vi "TCC_LIBRA.vi"() -> ()   [LabVIEW 2010]
doc: "Use this template to build a standard state machine design pattern. Each state executes code and determines which state to transition to. Contrast this design pattern with the User Interface Event Handler pattern, in which code executes in response to user actions. Contrast this design pattern also with the Queued Message Handler pattern, in which each message handling code can queue zero or more new messages."
uses:
  LV/TCC_03_02_2016/TCC_01_02_15.ctl
  <vilib>/Instr/_visa.llb/VISA Configure Serial Port (Instr).vi
  <vilib>/Utility/file.llb/Write To Spreadsheet File (DBL).vi
  <vilib>/Analysis/NI_AALBase.lvlib
panel:
  in  "port":u16=20551
  out "Resulting string (W)":string
  in  "COM PIC":refnum<visa-resource-name>
  in  "Quit":bool
  in  "Inicia Controle":bool
  out "Ajuste Fino":bool
  out "Ajuste Grosso":bool
  out "Quantidade de Passos N-1":sgl
  out "Medida N-1 (W)":dbl=0.027000000700354576 min=0.027000000700354576 max=0.27000001072883606 step=0.0005000000237487257 format="%0.8f"
  out "Diferença em %":dbl
  in  "Potência max Laser":dbl=0.001 min=0.001 max=0.3 step=0.0001
  out "Mínima Pot":dbl=0.009
  out "Meter Serial Number 5":string
  in  "Location of FieldMax2Lib.dll in 5":path=path "C:/Windows/System32/FieldMax2Lib.dll"
  out "Meter Serial Number 4":string
  in  "Location of FieldMax2Lib.dll in 4":path=path "C:/Windows/System32/FieldMax2Lib.dll"
  out "Meter Serial Number 3":string
  out "Motor Sensor":bool
  out "Motor Disco":bool
  out "Shutter ON (Verde_Claro)/ OFF (Verde_Escuro)":bool
  out "Measurement (W)":dbl format="%0.8f"
  out "Desv.Padrão":dbl format="%.8f"
  out "Quantidade de Passos":sgl
  in  "Média (W)":dbl=0.027000000700354576 min=0.027000000700354576 max=0.27000001072883606 step=0.0005000000237487257 format="%0.8f"
  in  "Setpoint (W)":dbl=0.027000000700354576 min=0.027000000700354576 max=0.27000001072883606 step=0.0005000000237487257
  out "Coef. Inicial":dbl
  out "i":i32
  out "DeltaP":dbl
  out "Coeficiente novo":dbl
  out "Inicia\nAutomático":bool
  in  "Mensagem de erro renviada":string
  out "Máxima Pot":dbl=0.145
  in  "service name":string="localhost"
  out "FS/AS?":string
  out "connection P3D ID out":refnum<k5>
  out "Erro TCP 3DP":errorcluster
  out "Erro comando PIC":errorcluster
  in  "Location of FieldMax2Lib.dll in 3":path=path "C:/Windows/System32/FieldMax2Lib.dll"
  out "Comandos para o PIC":string
  out "return count":u32
  out "data out":string
  out "bytes written":i32
  out "Loop":i32
  out "initialized array":sgl[](array[numeric]) format="%#_8g"
  out "N_passos string":string
  # "- Entradas do programa:"
  # "- Informações do medidor:"
  # "-Indicadores:"
  # "- Variáveis auxiliares:"
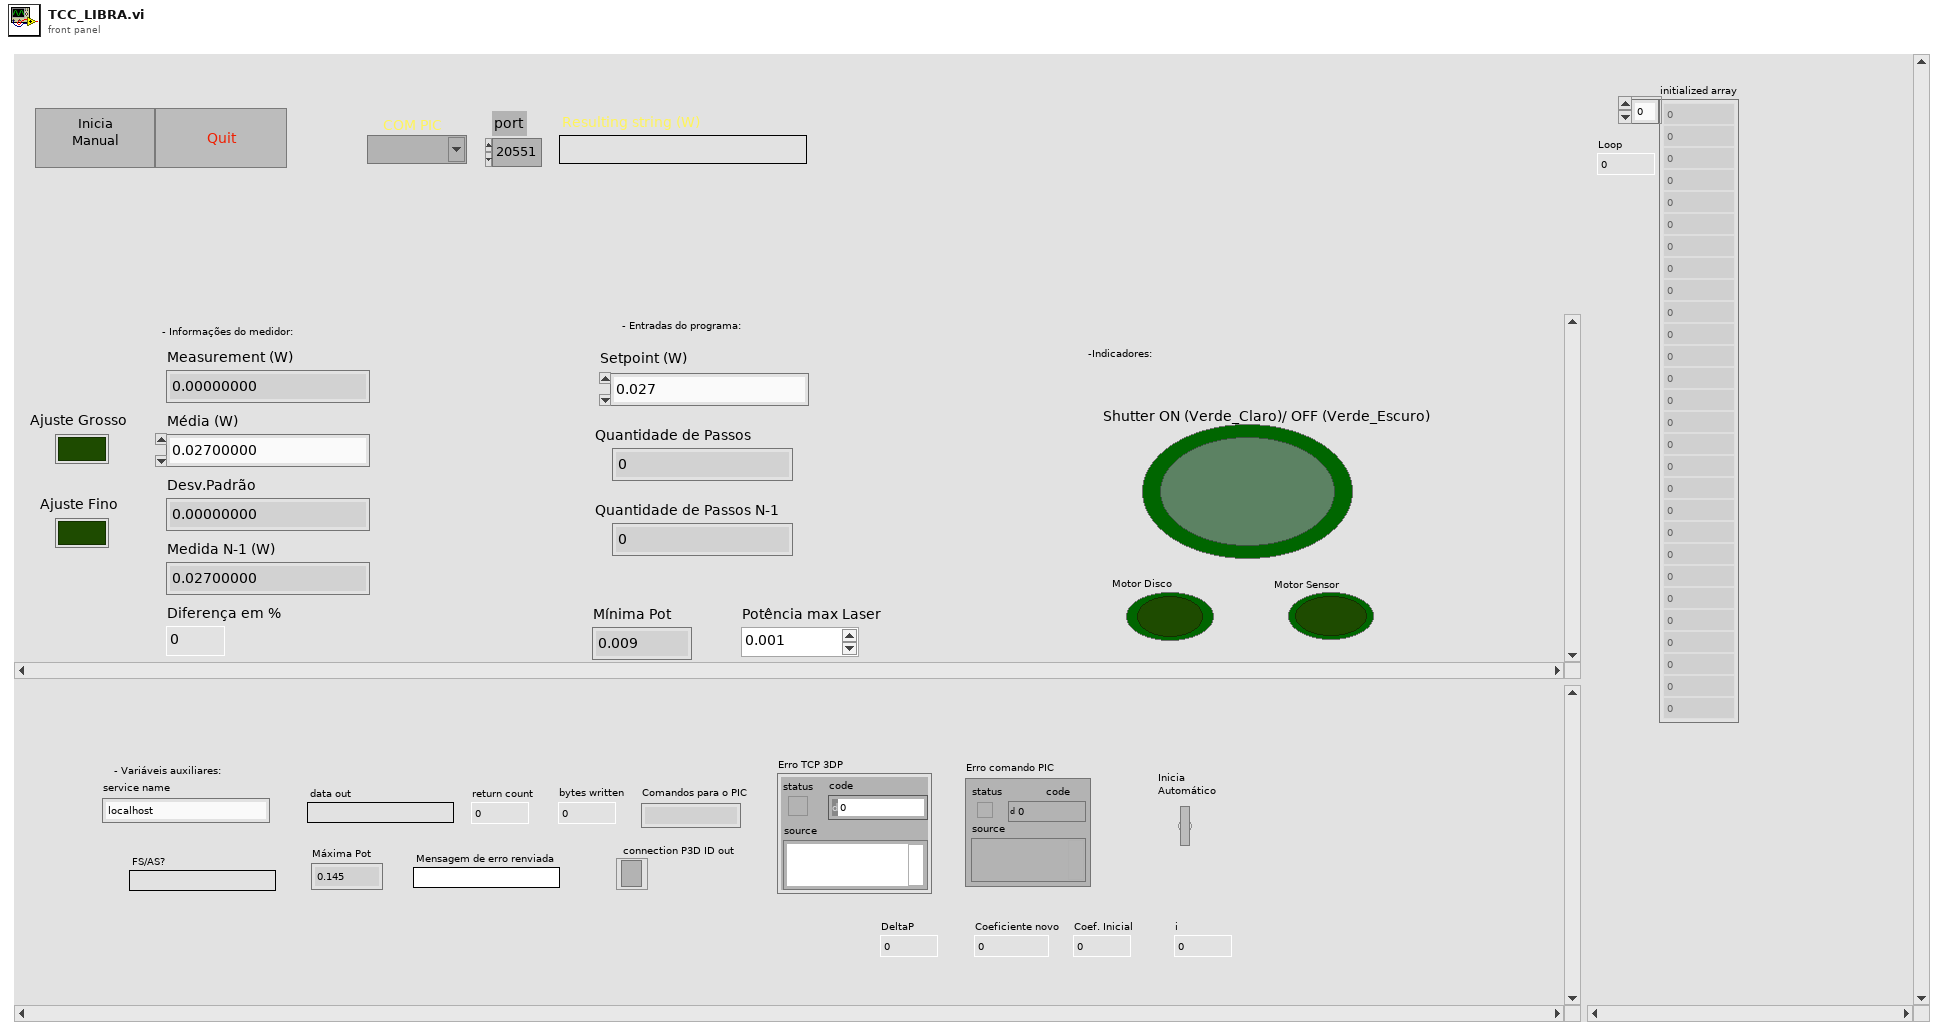
[diagram p1: front panel]
types:
  T1 = typedef "TCC_01_02_15.ctl" = enum16{"Receber Potencia", "Eventos", "Limites_P3D", "Apenas Shutter", "Ajuste de Potência", "Stop"}
  T2 = enum8{"Enabled", "Disabled", "Disabled and Grayed Out"}
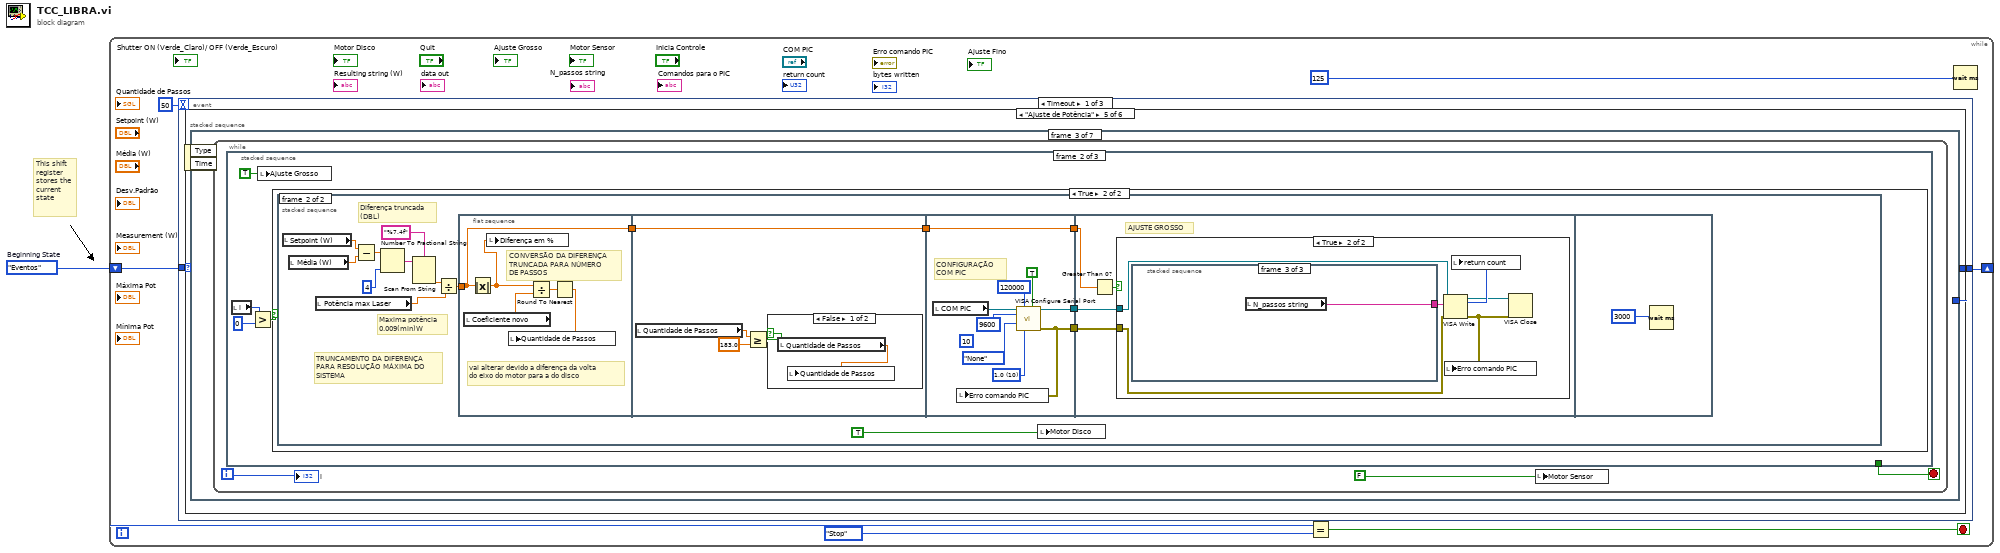
[diagram p0: block diagram]
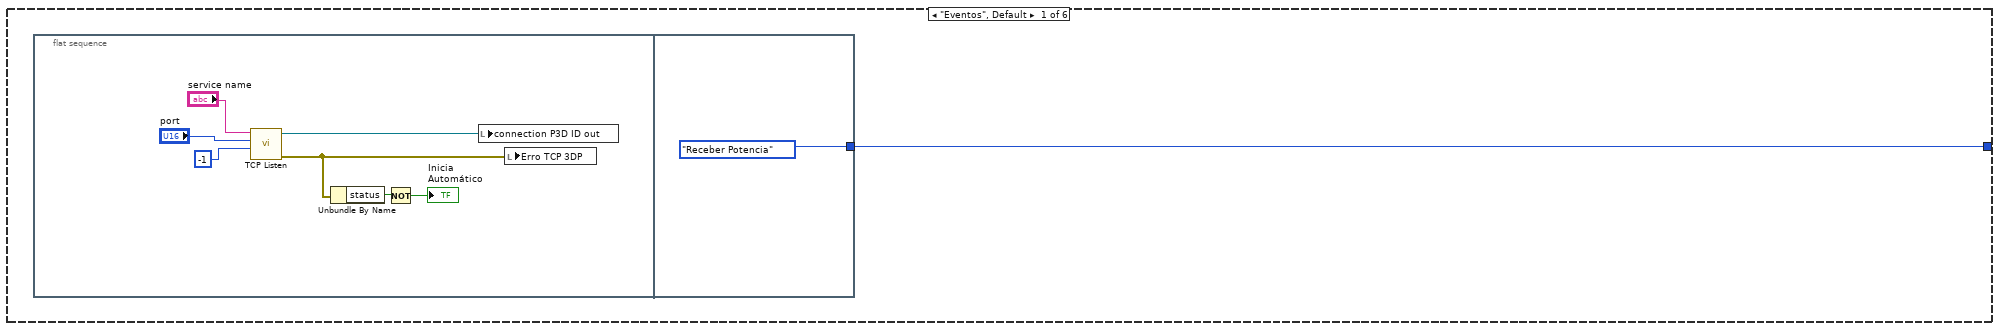
[diagram p2: hidden frame]
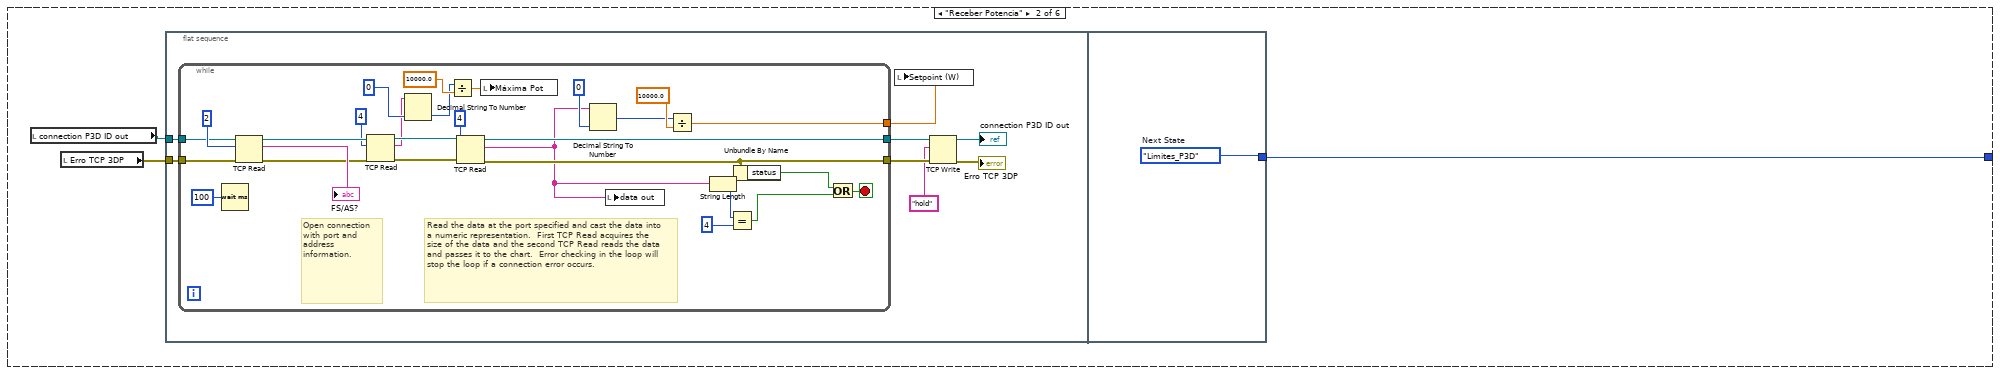
[diagram p3: hidden frame]
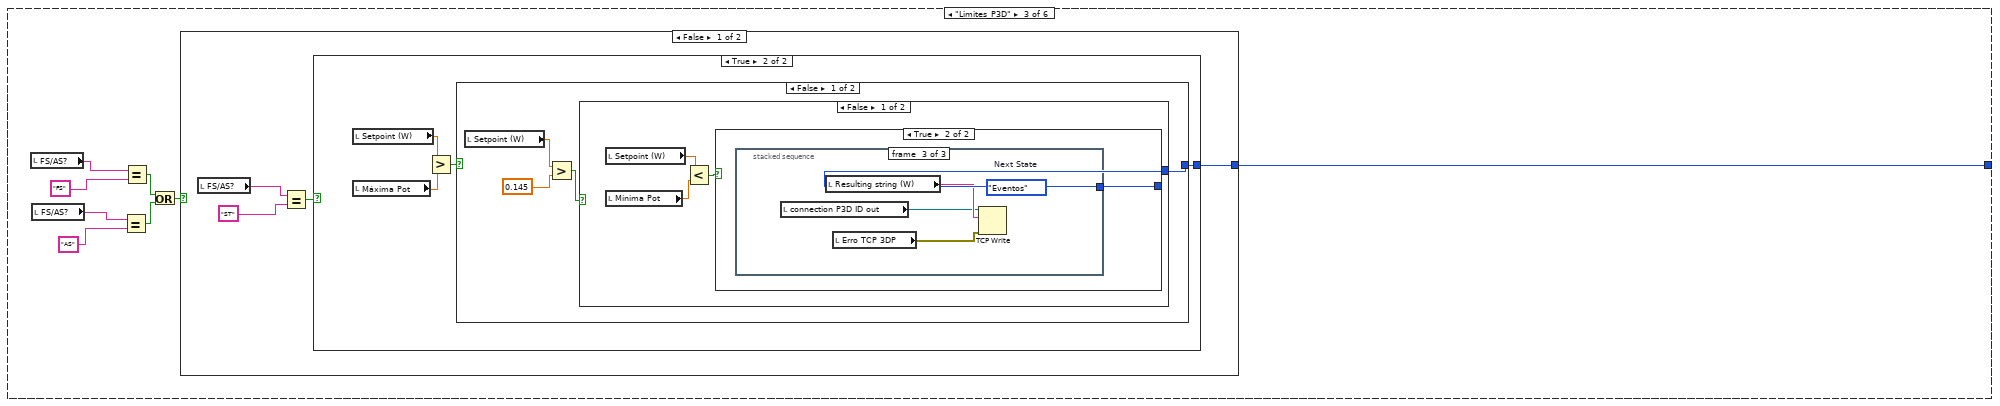
[diagram p4: hidden frame]
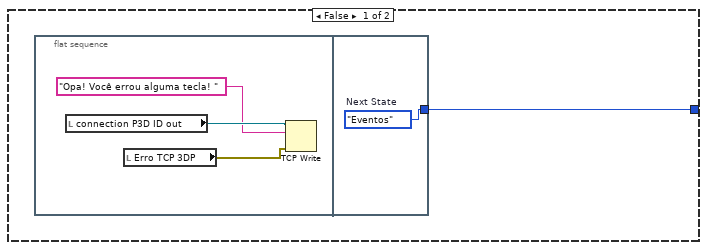
[diagram p5: hidden frame]
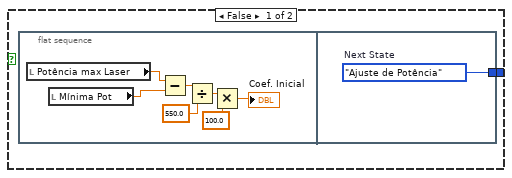
[diagram p6: hidden frame]
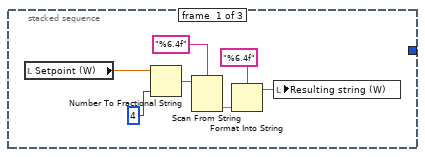
[diagram p7: hidden frame]
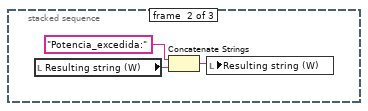
[diagram p8: hidden frame]
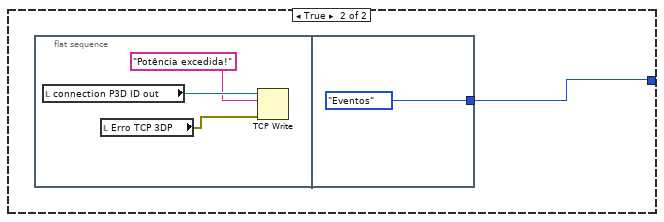
[diagram p9: hidden frame]
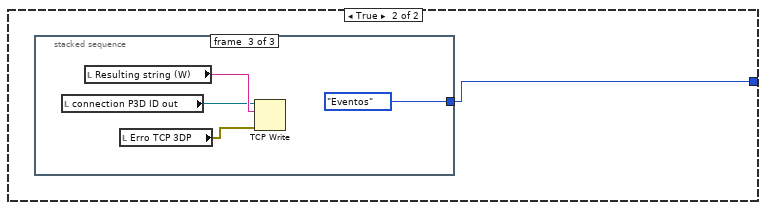
[diagram p10: hidden frame]
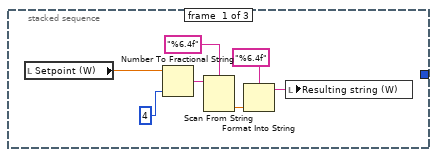
[diagram p11: hidden frame]
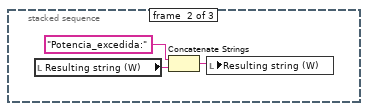
[diagram p12: hidden frame]
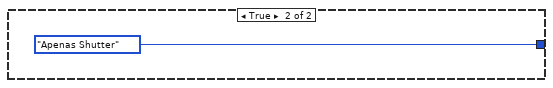
[diagram p13: hidden frame]
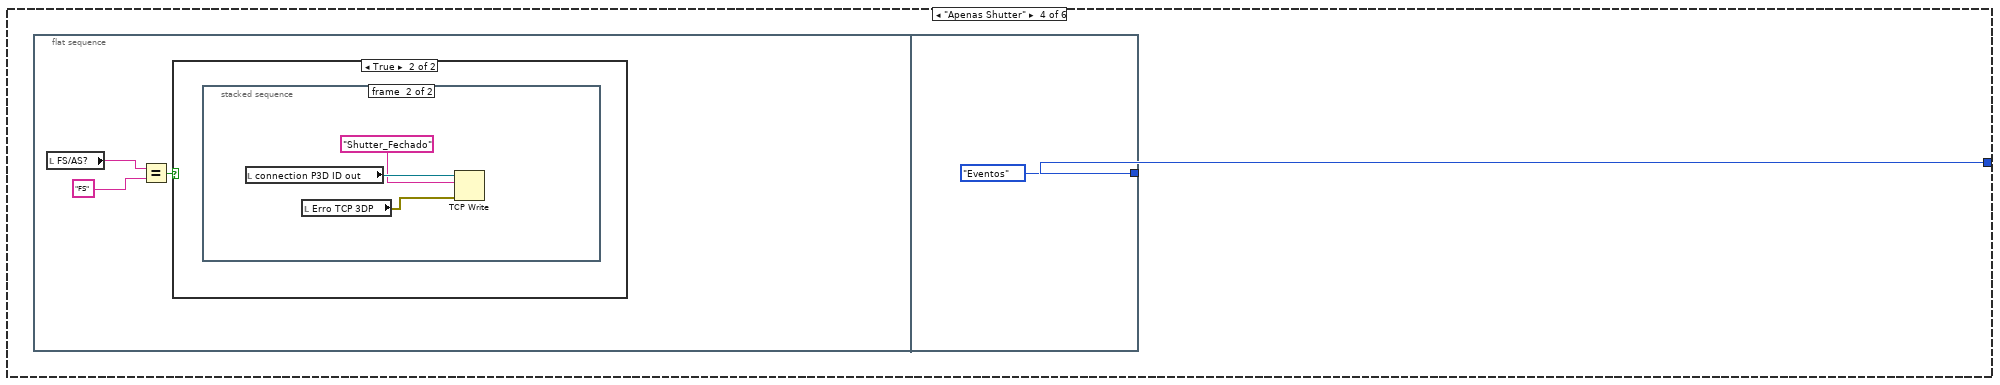
[diagram p14: hidden frame]
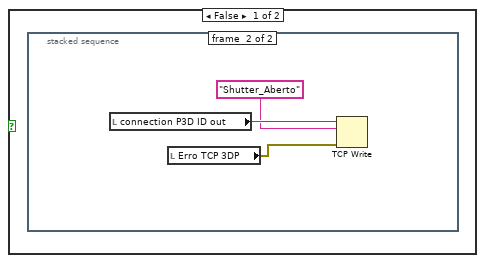
[diagram p15: hidden frame]
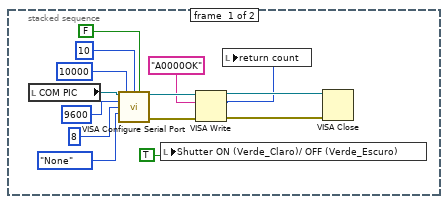
[diagram p16: hidden frame]
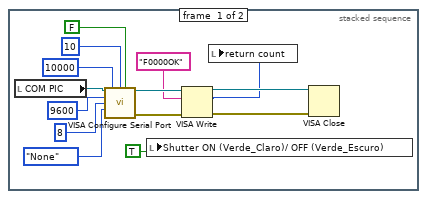
[diagram p17: hidden frame]
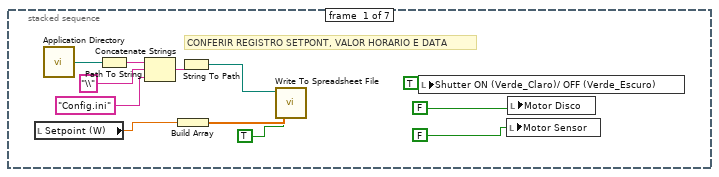
[diagram p18: hidden frame]
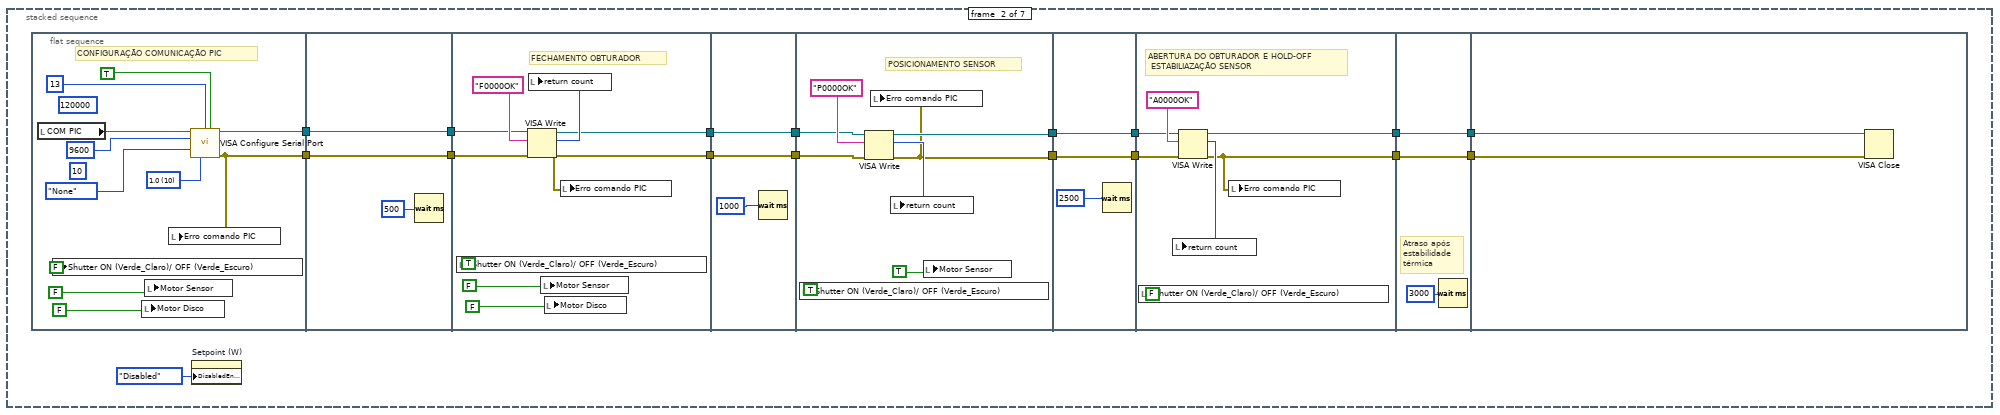
[diagram p19: hidden frame]
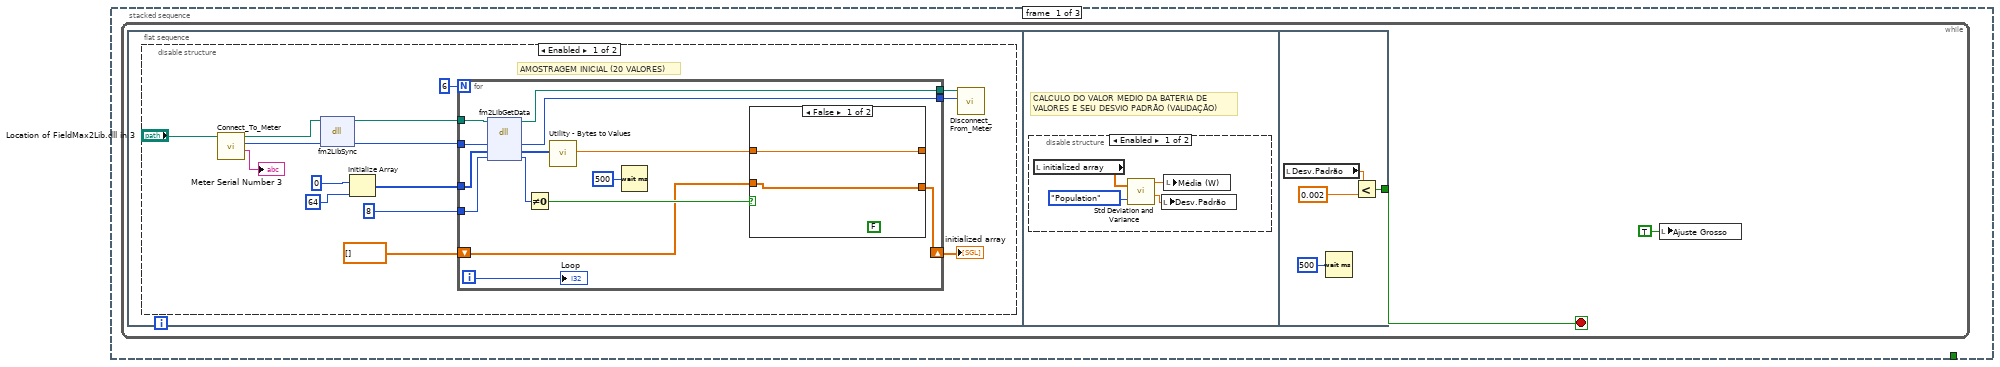
[diagram p20: hidden frame]
diagram:
  w1 = TCC_01_02_15."Eventos"  # Beginning State
  # "This shift\nregister\nstores the\ncurrent\nstate"
  n1 = while {
    shift-right: [w4] -> _
    shift-left: w1 -> [w5]
    stop <- w7 stop-if-true
    n2 = event shown="[0] Timeout" {
      selector: _ -> [_ _ _]
      dyn-events: _ -> [_ _ _]
      timeout: 50 -> [_ _ _]
      tunnel: w5 -> [w9 _ _]
      tunnel: [w8 w713 TCC_01_02_15."Stop" ("States")] -> w4
      event Timeout {
        n3 = event-data() -> ()  [unwired: 1 in, 2 out]
        n4 = case shown="\"Ajuste de Potência\"" w9 {
          tunnel: [w10 w21 w66 w133 w172 TCC_01_02_15."Eventos" ("Next State")] -> w8
          frame "Eventos", Default {
            n5 = flat-sequence {
              tunnel: [TCC_01_02_15."Receber Potencia" ("States")] -> w10
              frame #0 {
                n6 = call <vilib>:"TCP Listen.vi"("timeout ms (wait forever: -1)"=-1, "port"="port", "service name"="service name") -> ("error out"=w12:errorcluster, "connection ID"=w11:refnum<k5>)  [unwired: 5 in, 2 out]
                n7 = Unbundle By Name(w12) -> ("status"=w14:bool)
                n8 = Not(x=w14) -> (.not. x?=→"Inicia\nAutomático":bool)
                n9 = local write "connection P3D ID out"(w11) -> ()
                n10 = local write "Erro TCP 3DP"(w12) -> ()
              }
              frame #1 {
              }
            }
          }
          frame "Receber Potencia" {
            n11 = local read "connection P3D ID out"() -> (w19:refnum<k5>)
            n12 = local read "Erro TCP 3DP"() -> (w20:errorcluster)
            n13 = flat-sequence {
              tunnel: w19 -> [w23]
              tunnel: w20 -> [w22]
              tunnel: [w58] -> w21
              frame #0 {
                n14 = while {
                  tunnel: [w46] -> w28
                  tunnel: [w47] -> w29
                  tunnel: w23 -> [w53]
                  tunnel: w22 -> [w52]
                  tunnel: [w51] -> w26
                  stop <- w40 stop-if-true
                  # "Read the data at the port specified and cast the data into a numeric representation.  First TCP Read acquires the size of the data and the second TCP Read reads the data and passes it to the chart.  Error checking in the loop will stop the loop if a connection error occurs."
                  # "Open connection\nwith port and \naddress information."
                  n15 = Wait (ms)(milliseconds to wait=u32 100) -> ()  [unwired: 1 out]
                  n16 = TCP Read(connection ID=w53, bytes to read=2, error in (no error)=w52) -> (connection ID out=w38:refnum<k5>, data out=→"FS/AS?":string, error out=w39:errorcluster)  [unwired: 2 in]
                  n17 = TCP Read(connection ID=w38, bytes to read=4, error in (no error)=w39) -> (connection ID out=w37:refnum<k5>, data out=w34:string, error out=w36:errorcluster)  [unwired: 2 in]
                  n18 = Decimal String To Number(string=w34, default (0L)=0 ("default (0 I32)")) -> (number=w32:i32)  [unwired: 1 in, 1 out]
                  n19 = Divide(x=w32, y=10000.0) -> (x/y=w31:dbl)
                  n20 = TCP Read(connection ID=w37, bytes to read=u32 4, error in (no error)=w36) -> (connection ID out=w47:refnum<k5>, data out=w42:string, error out=w46:errorcluster)  [unwired: 2 in]
                  n21 = local write "Máxima Pot"(w31) -> ()
                  n22 = Decimal String To Number(string=w42, default (0L)=u32 0 ("default (0 I32)")) -> (number=w44:u32)  [unwired: 1 in, 1 out]
                  n23 = local write "data out"(w42) -> ()
                  n24 = Divide(x=w44, y=10000.0) -> (x/y=w51:dbl)
                  n25 = String Length(string=w42) -> (length=w43:i32)
                  n26 = Equal?(x=w43, y=4) -> (x = y?=w49:bool)
                  n27 = Unbundle By Name(w46) -> ("status"=w57:bool)
                  n28 = Or(x=w57, y=w49) -> (x .or. y?=w40:bool)
                }
                n29 = local write "Setpoint (W)"(w26) -> ()
                n30 = TCP Write(connection ID=w29, data in="hold", error in (no error)=w28) -> (connection ID out=→"connection P3D ID out":refnum<k5>, error out=→"Erro TCP 3DP":errorcluster)  [unwired: 1 in, 1 out]
              }
              frame #1 {
                w58 = TCC_01_02_15."Limites_P3D"  # Next State
              }
            }
          }
          frame "Limites_P3D" {
            n31 = local read "FS/AS?"() -> (w59:string)
            n32 = local read "FS/AS?"() -> (w60:string)
            n33 = Equal?(x=w60, y="AS") -> (x = y?=w62:bool)
            n34 = Equal?(x=w59, y="FS") -> (x = y?=w64:bool)
            n35 = Or(x=w64, y=w62) -> (x .or. y?=w61:bool)
            n36 = case shown="False" w61 {
              tunnel: [w70 TCC_01_02_15."Apenas Shutter" ("States")] -> w66
              frame False {
                n37 = local read "FS/AS?"() -> (w69:string)
                n38 = Equal?(x=w69, y="ST") -> (x = y?=w67:bool)
                n39 = case shown="True" w67 {
                  tunnel: [w71 w76] -> w70
                  frame False {
                    n40 = flat-sequence {
                      tunnel: [w75] -> w71
                      frame #0 {
                        n41 = local read "connection P3D ID out"() -> (w74:refnum<k5>)
                        n42 = local read "Erro TCP 3DP"() -> (w73:errorcluster)
                        n43 = TCP Write(connection ID=w74, data in="Opa! Você errou alguma tecla! ", error in (no error)=w73) -> ()  [unwired: 1 in, 3 out]
                      }
                      frame #1 {
                        w75 = TCC_01_02_15."Eventos"  # Next State
                      }
                    }
                  }
                  frame True {
                    n44 = local read "Setpoint (W)"() -> (w78:dbl)
                    n45 = local read "Máxima Pot"() -> (w79:dbl)
                    n46 = Greater?(x=w78, y=w79) -> (0:w77:bool)
                    n47 = case shown="False" w77 {
                      tunnel: [w83 w117] -> w76
                      frame False {
                        n48 = local read "Setpoint (W)"() -> (w81:dbl)
                        n49 = Greater?(x=w81, y=0.145) -> (0:w80:bool)
                        n50 = case shown="False" w80 {
                          tunnel: [w84 w112] -> w83
                          frame False {
                            n51 = local read "Setpoint (W)"() -> (w87:dbl)
                            n52 = local read "Mínima Pot"() -> (w86:dbl)
                            n53 = Less?(x=w87, y=w86) -> (x < y?=w85:bool)
                            n54 = case shown="True" w85 {
                              tunnel: [w88 w97] -> w84
                              frame False {
                                n55 = flat-sequence {
                                tunnel: [w96] -> w88
                                frame #0 {
                                n56 = local read "Potência max Laser"() -> (w94:dbl)
                                n57 = local read "Mínima Pot"() -> (w95:dbl)
                                n58 = Subtract(x=w94, y=w95) -> (x-y=w93:dbl)
                                n59 = Divide(x=w93, y=550.0) -> (x/y=w91:dbl)
                                n60 = Multiply(x=w91, y=100.0) -> (x*y=→"Coef. Inicial":dbl)
                                }
                                frame #1 {
                                w96 = TCC_01_02_15."Ajuste de Potência"  # Next State
                                }
                                }
                              }
                              frame True {
                                n61 = stacked-sequence {
                                tunnel: [_ _ w110] -> w97
                                frame #0 {
                                n62 = local read "Setpoint (W)"() -> (w101:dbl)
                                n63 = Number To Fractional String(number=w101, precision (6)=i16 4) -> (F-format string=w102:string)  [unwired: 2 in]
                                n64 = Scan From String(format string="%6.4f", input string=w102) -> (output 1=w98:dbl)  [unwired: 3 in, 3 out]
                                n65 = Format Into String(format string="%6.4f", w98) -> (resulting string=w99:string)  [unwired: 2 in, 1 out]
                                n66 = local write "Resulting string (W)"(w99) -> ()
                                }
                                frame #1 {
                                n67 = local read "Resulting string (W)"() -> (w107:string)
                                n68 = Concatenate Strings("Potencia_excedida:", w107) -> (w105:string)
                                n69 = local write "Resulting string (W)"(w105) -> ()
                                }
                                frame #2 {
                                w110 = TCC_01_02_15."Eventos"  # Next State
                                n70 = local read "connection P3D ID out"() -> (w109:refnum<k5>)
                                n71 = local read "Resulting string (W)"() -> (w111:string)
                                n72 = local read "Erro TCP 3DP"() -> (w108:errorcluster)
                                n73 = TCP Write(connection ID=w109, data in=w111, error in (no error)=w108) -> ()  [unwired: 1 in, 3 out]
                                }
                                }
                              }
                            }
                          }
                          frame True {
                            n74 = flat-sequence {
                              tunnel: [TCC_01_02_15."Eventos" ("States")] -> w112
                              frame #0 {
                                n75 = local read "connection P3D ID out"() -> (w114:refnum<k5>)
                                n76 = local read "Erro TCP 3DP"() -> (w115:errorcluster)
                                n77 = TCP Write(connection ID=w114, data in="Potência excedida!", error in (no error)=w115) -> ()  [unwired: 1 in, 3 out]
                              }
                              frame #1 {
                              }
                            }
                          }
                        }
                      }
                      frame True {
                        n78 = stacked-sequence {
                          tunnel: [_ _ TCC_01_02_15."Eventos" ("States")] -> w117
                          frame #0 {
                            n79 = local read "Setpoint (W)"() -> (w121:dbl)
                            n80 = Number To Fractional String(number=w121, precision (6)=i16 4) -> (F-format string=w122:string)  [unwired: 2 in]
                            n81 = Scan From String(format string="%6.4f", input string=w122) -> (output 1=w118:dbl)  [unwired: 3 in, 3 out]
                            n82 = Format Into String(format string="%6.4f", w118) -> (resulting string=w119:string)  [unwired: 2 in, 1 out]
                            n83 = local write "Resulting string (W)"(w119) -> ()
                          }
                          frame #1 {
                            n84 = local read "Resulting string (W)"() -> (w127:string)
                            n85 = Concatenate Strings("Potencia_excedida:", w127) -> (w125:string)
                            n86 = local write "Resulting string (W)"(w125) -> ()
                          }
                          frame #2 {
                            n87 = local read "connection P3D ID out"() -> (w128:refnum<k5>)
                            n88 = local read "Resulting string (W)"() -> (w131:string)
                            n89 = local read "Erro TCP 3DP"() -> (w129:errorcluster)
                            n90 = TCP Write(connection ID=w128, data in=w131, error in (no error)=w129) -> ()  [unwired: 1 in, 3 out]
                          }
                        }
                      }
                    }
                  }
                }
              }
              frame True {
              }
            }
          }
          frame "Apenas Shutter" {
            n91 = flat-sequence {
              tunnel: [TCC_01_02_15."Eventos" ("States")] -> w133
              frame #0 {
                n92 = local read "FS/AS?"() -> (w136:string)
                n93 = Equal?(x=w136, y="FS") -> (x = y?=w134:bool)
                n94 = case shown="True" w134 {
                  frame False {
                    n95 = stacked-sequence {
                      frame #0 {
                        n96 = local read "COM PIC"() -> (w143:refnum<visa-resource-name>)
                        n97 = call-poly "VISA Configure Serial Port"("VISA resource name"=w143, "timeout (10sec)"=u32 10000, "termination char\n(0xA = '\\n' = LF)"=u8 10 ("termination char\n(0xA = '\\n' = LF)"), "Enable Termination\nChar (T)"=FALSE ("Enable Termination\nChar (T)"), "baud rate (9600)"=u32 9600, "data bits (8)"=u16 8, "parity (0:none)"=enum16{"None", "Odd", "Even", "Mark", "Space"}."None") -> ("VISA resource name out"=w142:refnum<visa-resource-name>, "error out"=w141:errorcluster)  [unwired: 7 in]
                        n98 = local write "Shutter ON (Verde_Claro)/ OFF (Verde_Escuro)"(TRUE ("Inicia Controle")) -> ()
                        n99 = VISA Write(VISA resource name=w142, write buffer="A0000OK", error in (no error)=w141) -> (VISA resource name out=w138:refnum<visa-resource-name>, return count=w137:u32, error out=w139:errorcluster)
                        n100 = local write "return count"(w137) -> ()
                        n101 = VISA Close(VISA resource name=w138, error in (no error)=w139) -> ()  [unwired: 1 out]
                      }
                      frame #1 {
                        n102 = local read "connection P3D ID out"() -> (w152:refnum<k5>)
                        n103 = local read "Erro TCP 3DP"() -> (w153:errorcluster)
                        n104 = TCP Write(connection ID=w152, data in="Shutter_Aberto", error in (no error)=w153) -> ()  [unwired: 1 in, 3 out]
                      }
                    }
                  }
                  frame True {
                    n105 = stacked-sequence {
                      frame #0 {
                        n106 = local read "COM PIC"() -> (w160:refnum<visa-resource-name>)
                        n107 = call-poly "VISA Configure Serial Port"("VISA resource name"=w160, "timeout (10sec)"=u32 10000, "termination char\n(0xA = '\\n' = LF)"=u8 10 ("termination char\n(0xA = '\\n' = LF)"), "Enable Termination\nChar (T)"=FALSE ("Enable Termination\nChar (T)"), "baud rate (9600)"=u32 9600, "data bits (8)"=u16 8, "parity (0:none)"=enum16{"None", "Odd", "Even", "Mark", "Space"}."None") -> ("VISA resource name out"=w159:refnum<visa-resource-name>, "error out"=w158:errorcluster)  [unwired: 7 in]
                        n108 = local write "Shutter ON (Verde_Claro)/ OFF (Verde_Escuro)"(TRUE ("Inicia Controle")) -> ()
                        n109 = VISA Write(VISA resource name=w159, write buffer="F0000OK", error in (no error)=w158) -> (VISA resource name out=w155:refnum<visa-resource-name>, return count=w154:u32, error out=w156:errorcluster)
                        n110 = local write "return count"(w154) -> ()
                        n111 = VISA Close(VISA resource name=w155, error in (no error)=w156) -> ()  [unwired: 1 out]
                      }
                      frame #1 {
                        n112 = local read "connection P3D ID out"() -> (w169:refnum<k5>)
                        n113 = local read "Erro TCP 3DP"() -> (w170:errorcluster)
                        n114 = TCP Write(connection ID=w169, data in="Shutter_Fechado", error in (no error)=w170) -> ()  [unwired: 1 in, 3 out]
                      }
                    }
                  }
                }
              }
              frame #1 {
              }
            }
          }
          frame "Ajuste de Potência" {
            n115 = stacked-sequence {
              tunnel: [_ _ _ _ _ _ TCC_01_02_15."Eventos" ("States")] -> w172
              frame #0 {
                # "CONFERIR REGISTRO SETPONT, VALOR HORARIO E DATA"
                n116 = local read "Setpoint (W)"() -> (w177:dbl)
                n117 = call <vilib>:"Application Directory.vi"() -> ("Application Directory"=w184:path)
                n118 = Path To String(path=w184) -> (string=w182:string)
                n119 = Concatenate Strings(w182, "\\" ("string"), "Config.ini" ("replace string (\"\")")) -> (w183:string)
                n120 = Build Array(w177) -> (w180:dbl[])
                n121 = String To Path(string=w183) -> (path=w181:path)
                n122 = call-poly <vilib>:"Write To Spreadsheet File.vi"("append to file? (new file:F)"=TRUE, "1D data"=w180, "file path (dialog if empty)"=w181) -> ()  [unwired: 5 in, 1 out]
                n123 = local write "Shutter ON (Verde_Claro)/ OFF (Verde_Escuro)"(TRUE) -> ()
                n124 = local write "Motor Sensor"(FALSE) -> ()
                n125 = local write "Motor Disco"(FALSE) -> ()
              }
              frame #1 {
                n126 = flat-sequence {
                  tunnel: [w204] -> w196
                  tunnel: [w202] -> w194
                  tunnel: w196 -> [w215]
                  tunnel: [w215] -> w195
                  tunnel: w194 -> [w214]
                  tunnel: [w214] -> w193
                  tunnel: w195 -> [w218]
                  tunnel: w193 -> [w219]
                  tunnel: [w217] -> w188
                  tunnel: [w216] -> w186
                  tunnel: w188 -> [w227]
                  tunnel: [w227] -> w187
                  tunnel: w186 -> [w226]
                  tunnel: [w226] -> w185
                  tunnel: w187 -> [w231]
                  tunnel: w185 -> [w230]
                  tunnel: [w229] -> w192
                  tunnel: [w228] -> w190
                  tunnel: w192 -> [w238]
                  tunnel: [w238] -> w191
                  tunnel: w190 -> [w237]
                  tunnel: [w237] -> w189
                  tunnel: w191 -> [w242]
                  tunnel: w189 -> [w241]
                  tunnel: [w240] -> w199
                  tunnel: [w239] -> w197
                  tunnel: [w247] -> w200
                  tunnel: w199 -> [w247]
                  tunnel: [w246] -> w198
                  tunnel: w197 -> [w246]
                  tunnel: w200 -> [w250]
                  tunnel: w198 -> [w249]
                  frame #0 {
                    w203 = u16 10 items=["1.0"=10, "1.5"=15, "2.0"=20] ("stop bits (10: 1 bit)")
                    (unwired) u32 120000 ("timeout (10sec)")
                    (unwired) u16 10 ("data bits (8)")
                    # "CONFIGURAÇÃO COMUNICAÇÃO PIC"
                    n127 = local read "COM PIC"() -> (w212:refnum<visa-resource-name>)
                    n128 = local write "Shutter ON (Verde_Claro)/ OFF (Verde_Escuro)"(FALSE ("Inicia Controle")) -> ()
                    n129 = local write "Motor Disco"(FALSE) -> ()
                    n130 = local write "Motor Sensor"(FALSE) -> ()
                    n131 = call-poly "VISA Configure Serial Port"("VISA resource name"=w212, "termination char\n(0xA = '\\n' = LF)"=u8 13 ("termination char\n(0xA = '\\n' = LF)"), "Enable Termination\nChar (T)"=TRUE, "baud rate (9600)"=u32 9600, "parity (0:none)"=enum16{"None", "Odd", "Even", "Mark", "Space"}."None", "stop bits (10: 1 bit)"=w203) -> ("VISA resource name out"=w204:refnum<visa-resource-name>, "error out"=w202:errorcluster)  [unwired: 8 in]
                    n132 = local write "Erro comando PIC"(w202) -> ()
                  }
                  frame #1 {
                    n133 = Wait (ms)(milliseconds to wait=500) -> ()  [unwired: 1 out]
                  }
                  frame #2 {
                    # "FECHAMENTO OBTURADOR"
                    n134 = local write "Shutter ON (Verde_Claro)/ OFF (Verde_Escuro)"(TRUE) -> ()
                    n135 = VISA Write(VISA resource name=w218, write buffer="F0000OK", error in (no error)=w219) -> (VISA resource name out=w217:refnum<visa-resource-name>, return count=w223:u32, error out=w216:errorcluster)
                    n136 = local write "return count"(w223) -> ()
                    n137 = local write "Motor Sensor"(FALSE) -> ()
                    n138 = local write "Motor Disco"(FALSE) -> ()
                    n139 = local write "Erro comando PIC"(w216) -> ()
                  }
                  frame #3 {
                    n140 = Wait (ms)(milliseconds to wait=u32 1000) -> ()  [unwired: 1 out]
                  }
                  frame #4 {
                    # "POSICIONAMENTO SENSOR"
                    n141 = local write "Shutter ON (Verde_Claro)/ OFF (Verde_Escuro)"(TRUE) -> ()
                    n142 = VISA Write(VISA resource name=w231, write buffer="P0000OK", error in (no error)=w230) -> (VISA resource name out=w229:refnum<visa-resource-name>, return count=w235:u32, error out=w228:errorcluster)
                    n143 = local write "Erro comando PIC"(w228) -> ()
                    n144 = local write "return count"(w235) -> ()
                    n145 = local write "Motor Sensor"(TRUE) -> ()
                  }
                  frame #5 {
                    n146 = Wait (ms)(milliseconds to wait=u32 2500) -> ()  [unwired: 1 out]
                  }
                  frame #6 {
                    # "ABERTURA DO OBTURADOR E HOLD-OFF\n ESTABILIAZAÇÃO SENSOR"
                    n147 = local write "Shutter ON (Verde_Claro)/ OFF (Verde_Escuro)"(FALSE) -> ()
                    n148 = VISA Write(VISA resource name=w242, write buffer="A0000OK", error in (no error)=w241) -> (VISA resource name out=w240:refnum<visa-resource-name>, return count=w245:u32, error out=w239:errorcluster)
                    n149 = local write "return count"(w245) -> ()
                    n150 = local write "Erro comando PIC"(w239) -> ()
                  }
                  frame #7 {
                    # "Atraso após\nestabilidade\ntérmica"
                    n151 = Wait (ms)(milliseconds to wait=u32 3000) -> ()  [unwired: 1 out]
                  }
                  frame #8 {
                    n152 = VISA Close(VISA resource name=w250, error in (no error)=w249) -> ()  [unwired: 1 out]
                  }
                }
                n153 = property on="Setpoint (W)" class="DigNum (strict)"("DisabledEnum"=T2."Disabled" ("Disabled")) -> ()  [unwired: 2 in, 2 out]
              }
              frame #2 {
                n154 = while {
                  i -> [w252]
                  stop <- w253 stop-if-true
                  n155 = stacked-sequence {
                    tunnel: [_ _ w494] -> w253
                    frame #0 {
                      n156 = while {
                        stop <- w255 stop-if-true
                        n157 = flat-sequence {
                          tunnel: [w297] -> w255
                          frame #0 {
                            n158 = disable-structure shown="Enabled" {
                              frame Enabled {
                                # "AMOSTRAGEM INICIAL (20 VALORES)"
                                n159 = call "Connect_To_Meter.vi"("Location of FieldMax2Lib.dll in"="Location of FieldMax2Lib.dll in 3") -> ("Meter Serial Number"=→"Meter Serial Number 3":string, "Meter ID out"=w258:i32, "Location of FieldMax2Lib.dll out"=w259:path)  [unwired: 6 in]
                                n160 = dll-call lib="C:/Windows/System32/FieldMax2Lib.dll" fn="fm2LibSync" label="Sync"(path in=w259, "h"=w258) -> (path out=w257:path, "h"=w256:i32)  [unwired: 3 in, 1 out]
                                n161 = Initialize Array(u8 0 ("element"), 64 ("dimension size")) -> (w265:u8[])
                                n162 = for {
                                N: 6 -> [_]
                                tunnel: w256 -> [w274]
                                tunnel: w265 -> [w280]
                                tunnel: i16 8 ("count") -> [w279]
                                tunnel: [w276] -> w261
                                tunnel: w257 -> [w281]
                                tunnel: [w275] -> w260
                                shift-right: [w271] -> w269
                                shift-left: sgl[] [] -> [w272]
                                i -> [w273]
                                n163 = dll-call lib="C:/Windows/System32/FieldMax2Lib.dll" fn="fm2LibGetData" label="Get Data"(path in=w281, "h"=w274, "returnBuffer"=w280, "count"=w279) -> (path out=w275:path, "h"=w276:i32, "returnBuffer"=w277:u8[], "count"=w278:i16)  [unwired: 3 in, 1 out]
                                n164 = Not Equal To 0?(x=w278) -> (x != 0?=w282:bool)
                                n165 = call "Utility - Bytes to Values.vi"("DataBuffer"=w277) -> ("Measurement Value"=w283:sgl)  [unwired: 9 in, 1 out]
                                n166 = Wait (ms)(milliseconds to wait=u32 500) -> ()  [unwired: 1 out]
                                n167 = case shown="False" w282 {
                                tunnel: w283 -> [w286 w287]
                                tunnel: [w286 w287] -> _
                                tunnel: w272 -> [w285 w289]
                                tunnel: [w285 w288] -> w271
                                frame False {
                                (unwired) FALSE
                                }
                                frame True {
                                n168 = local write "Measurement (W)"(w287) -> ()
                                n169 = Build Array (concatenate)(w289, w287) -> (w288:sgl[])
                                }
                                }
                                "Loop" <- w273
                                }
                                "initialized array" <- w269
                                n170 = call "Disconnect_From_Meter.vi"("Location of FieldMax2Lib.dll in"=w260, "Meter ID in"=w261) -> ()  [unwired: 7 in, 2 out]
                              }
                              frame Disabled {
                                n171 = Wait (ms)(milliseconds to wait=u32 500) -> ()  [unwired: 1 out]
                                n172 = local write "Média (W)"(0.105 ("Measurement")) -> ()
                              }
                            }
                          }
                          frame #1 {
                            # "CALCULO DO VALOR MEDIO DA BATERIA DE\nVALORES E SEU DESVIO PADRÃO (VALIDAÇÃO)"
                            n173 = disable-structure shown="Enabled" {
                              frame Enabled {
                                n174 = local read "initialized array"() -> (w292:sgl[])
                                n175 = call <vilib>:"Std Deviation and Variance.vi"("X"=w292, "Weighting (Sample)"=enum16{"Sample", "Population"}."Population") -> ("mean"=w295:dbl, "standard deviation"=w294:dbl)  [unwired: 1 out]
                                n176 = local write "Desv.Padrão"(w294) -> ()
                                n177 = local write "Média (W)"(w295) -> ()
                              }
                              frame Disabled {
                              }
                            }
                          }
                          frame #2 {
                            n178 = local read "Desv.Padrão"() -> (w298:dbl)
                            n179 = Wait (ms)(milliseconds to wait=u32 500) -> ()  [unwired: 1 out]
                            n180 = Less?(x=w298, y=0.002) -> (x < y?=w297:bool)
                          }
                        }
                        n181 = local write "Ajuste Grosso"(TRUE ("Ajuste Grosso")) -> ()
                      }
                    }
                    frame #1 {
                      n182 = local read "i"() -> (w303:i32)
                      n183 = Greater?(x=w303, y=0) -> (0:w301:bool)
                      n184 = local write "Ajuste Grosso"(TRUE ("Ajuste Grosso")) -> ()
                      n185 = case shown="True" w301 {
                        frame False {
                          # "TRUNCAMENTO DA DIFERENÇA \nPARA RESOLUÇÃO MÁXIMA DO\nSISTEMA"
                          # "Maxima potência\n0.009(min)W"
                          # "Diferença truncada\n(DBL)"
                          n186 = local read "Setpoint (W)"() -> (w313:dbl)
                          n187 = local read "Média (W)"() -> (w312:dbl)
                          n188 = Subtract(x=w313, y=w312) -> (x-y=w306:dbl)
                          n189 = Number To Fractional String(number=w306, precision (6)=i16 4) -> (F-format string=w309:string)  [unwired: 2 in]
                          n190 = Scan From String(format string="%7.4f", input string=w309) -> (output 1=w310:dbl)  [unwired: 3 in, 3 out]
                          n191 = Divide(x=w310, y="Potência max Laser") -> (x/y=w305:dbl)
                          n192 = flat-sequence {
                            tunnel: w305 -> [w320]
                            tunnel: [w320] -> w317
                            tunnel: w317 -> [w331]
                            tunnel: [w331] -> w316
                            tunnel: [w325] -> w315
                            tunnel: [w323] -> w314
                            tunnel: w316 -> [w334]
                            tunnel: w315 -> [w333]
                            tunnel: w314 -> [w332]
                            frame #0 {
                              # "CONVERSÃO DA DIFERENÇA\nTRUNCADA PARA NÚMERO\nDE PASSOS"
                              # "vai alterar devido a diferença da volta \ndo eixo do motor para a do disco"
                              n193 = local read "Coef. Inicial"() -> (w318:dbl)
                              n194 = Absolute Value(x=w320) -> (abs(x)=w319:dbl)
                              "Diferença em %" <- w319
                              n195 = Divide(x=w319, y=w318) -> (x/y=w321:dbl)
                              n196 = Round To Nearest(number=w321) -> (nearest integer value=w322:dbl)
                              n197 = local write "Quantidade de Passos"(w322) -> ()
                            }
                            frame #1 {
                              w324 = u16 10 items=["1.0"=10, "1.5"=15, "2.0"=20] ("stop bits (10: 1 bit)")
                              (unwired) u16 10 ("data bits (8)")
                              # "CONFIGURAÇÃO \nCOM PIC"
                              n198 = local read "COM PIC"() -> (w326:refnum<visa-resource-name>)
                              n199 = call-poly "VISA Configure Serial Port"("VISA resource name"=w326, "timeout (10sec)"=u32 120000, "Enable Termination\nChar (T)"=TRUE, "baud rate (9600)"=u32 9600, "parity (0:none)"=enum16{"None", "Odd", "Even", "Mark", "Space"}."None", "stop bits (10: 1 bit)"=w324) -> ("VISA resource name out"=w325:refnum<visa-resource-name>, "error out"=w323:errorcluster)  [unwired: 8 in]
                              n200 = local write "Erro comando PIC"(w323) -> ()
                            }
                            frame #2 {
                              # "AJUSTE GROSSO"
                              n201 = Greater Than 0?(x=w334) -> (x > 0?=w335:bool)
                              n202 = case shown="True" w335 {
                                tunnel: w333 -> [w339 w363]
                                tunnel: w332 -> [w338 w364]
                                frame False {
                                n203 = stacked-sequence {
                                tunnel: [_ _ w360] -> w341
                                frame #0 {
                                n204 = local read "Quantidade de Passos"() -> (w342:sgl)
                                n205 = Format Into String(format string="%d", w342) -> (resulting string=w344:string)  [unwired: 2 in, 1 out]
                                n206 = String Length(string=w344) -> (length=w345:i32)
                                n207 = case shown="1, Default" w345 {
                                tunnel: w344 -> [w347 w350 w352 w355]
                                frame 1, Default {
                                n208 = Concatenate Strings("000" ("string"), w347) -> (w348:string)
                                n209 = local write "N_passos string"(w348) -> ()
                                }
                                frame 2 {
                                n210 = Concatenate Strings("00" ("string"), w350) -> (w349:string)
                                n211 = local write "N_passos string"(w349) -> ()
                                }
                                frame 3 {
                                n212 = Concatenate Strings("0" ("string"), w352) -> (w353:string)
                                n213 = local write "N_passos string"(w353) -> ()
                                }
                                frame 4 {
                                n214 = local write "N_passos string"(w355) -> ()
                                }
                                }
                                }
                                frame #1 {
                                # "adicionar letra"
                                n215 = local read "N_passos string"() -> (w357:string)
                                n216 = Concatenate Strings("D" ("string"), w357, "OK" ("string")) -> (w359:string)
                                n217 = local write "N_passos string"(w359) -> ()
                                }
                                frame #2 {
                                n218 = local read "N_passos string"() -> (w360:string)
                                }
                                }
                                n219 = VISA Write(VISA resource name=w339, write buffer=w341, error in (no error)=w338) -> (VISA resource name out=w337:refnum<visa-resource-name>, return count=w340:u32, error out=w336:errorcluster)
                                n220 = local write "Erro comando PIC"(w336) -> ()
                                n221 = local write "return count"(w340) -> ()
                                n222 = VISA Close(VISA resource name=w337, error in (no error)=w336) -> ()  [unwired: 1 out]
                                }
                                frame True {
                                n223 = stacked-sequence {
                                tunnel: [_ _ w385] -> w366
                                frame #0 {
                                n224 = local read "Quantidade de Passos"() -> (w367:sgl)
                                n225 = Format Into String(format string="%d", w367) -> (resulting string=w369:string)  [unwired: 2 in, 1 out]
                                n226 = String Length(string=w369) -> (length=w370:i32)
                                n227 = case shown="3" w370 {
                                tunnel: w369 -> [w371 w375 w377 w380]
                                frame 1, Default {
                                n228 = Concatenate Strings("000" ("string"), w371) -> (w373:string)
                                n229 = local write "N_passos string"(w373) -> ()
                                }
                                frame 2 {
                                n230 = Concatenate Strings("00" ("string"), w375) -> (w374:string)
                                n231 = local write "N_passos string"(w374) -> ()
                                }
                                frame 3 {
                                n232 = Concatenate Strings("0" ("string"), w377) -> (w378:string)
                                n233 = local write "N_passos string"(w378) -> ()
                                }
                                frame 4 {
                                n234 = local write "N_passos string"(w380) -> ()
                                }
                                }
                                }
                                frame #1 {
                                n235 = local read "N_passos string"() -> (w382:string)
                                n236 = Concatenate Strings("I" ("string"), w382, "OK" ("string")) -> (w384:string)
                                n237 = local write "N_passos string"(w384) -> ()
                                }
                                frame #2 {
                                n238 = local read "N_passos string"() -> (w385:string)
                                }
                                }
                                n239 = VISA Write(VISA resource name=w363, write buffer=w366, error in (no error)=w364) -> (VISA resource name out=w362:refnum<visa-resource-name>, return count=w365:u32, error out=w361:errorcluster)
                                n240 = local write "Erro comando PIC"(w361) -> ()
                                n241 = local write "return count"(w365) -> ()
                                n242 = VISA Close(VISA resource name=w362, error in (no error)=w361) -> ()  [unwired: 1 out]
                                }
                              }
                            }
                            frame #3 {
                              n243 = local read "Quantidade de Passos"() -> (→"Quantidade de Passos N-1":sgl)
                              n244 = local read "Média (W)"() -> (→"Medida N-1 (W)":dbl)
                            }
                            frame #4 {
                              n245 = Wait (ms)(milliseconds to wait=3000) -> ()  [unwired: 1 out]
                            }
                          }
                          n246 = local write "Motor Disco"(TRUE) -> ()
                        }
                        frame True {
                          n247 = stacked-sequence {
                            frame #0 {
                              n248 = flat-sequence {
                                frame #0 {
                                n249 = local read "Medida N-1 (W)"() -> (w391:dbl)
                                n250 = local read "Média (W)"() -> (w392:dbl)
                                n251 = Subtract(x=w391, y=w392) -> (x-y=w390:dbl)
                                n252 = Absolute Value(x=w390) -> (abs(x)=→"DeltaP":dbl)
                                }
                                frame #1 {
                                n253 = local read "Quantidade de Passos N-1"() -> (w397:sgl)
                                n254 = local read "DeltaP"() -> (w396:dbl)
                                n255 = Divide(x=w396, y=w397) -> (x/y=w395:dbl)
                                n256 = Multiply(x=w395, y=100.0) -> (x*y=→"Coeficiente novo":dbl)
                                }
                                frame #2 {
                                n257 = local read "Quantidade de Passos N-1"() -> (w399:sgl)
                                n258 = local read "Média (W)"() -> (w398:dbl)
                                n259 = local write "Medida N-1 (W)"(w398) -> ()
                                n260 = local write "Quantidade de Passos"(w399) -> ()
                                }
                              }
                            }
                            frame #1 {
                              # "TRUNCAMENTO DA DIFERENÇA \nPARA RESOLUÇÃO MÁXIMA DO\nSISTEMA"
                              # "Maxima potência\n0.009(min)W"
                              # "Diferença truncada\n(DBL)"
                              n261 = local read "Setpoint (W)"() -> (w410:dbl)
                              n262 = local read "Média (W)"() -> (w409:dbl)
                              n263 = local read "Potência max Laser"() -> (w411:dbl)
                              n264 = Subtract(x=w410, y=w409) -> (x-y=w403:dbl)
                              n265 = Number To Fractional String(number=w403, precision (6)=i16 4) -> (F-format string=w406:string)  [unwired: 2 in]
                              n266 = Scan From String(format string="%7.4f", input string=w406) -> (output 1=w407:dbl)  [unwired: 3 in, 3 out]
                              n267 = Divide(x=w407, y=w411) -> (x/y=w402:dbl)
                              n268 = flat-sequence {
                                tunnel: w402 -> [w417]
                                tunnel: [w417] -> w401
                                tunnel: w401 -> [w423]
                                tunnel: [w423] -> w400
                                tunnel: w400 -> [w434]
                                tunnel: [w434] -> w414
                                tunnel: [w428] -> w413
                                tunnel: [w426] -> w412
                                tunnel: w414 -> [w437]
                                tunnel: w413 -> [w436]
                                tunnel: w412 -> [w435]
                                frame #0 {
                                # "CONVERSÃO DA DIFERENÇA\nTRUNCADA PARA NÚMERO\nDE PASSOS"
                                # "vai alterar devido a diferença da volta \ndo eixo do motor para a do disco"
                                n269 = local read "Coeficiente novo"() -> (w416:dbl)
                                n270 = Absolute Value(x=w417) -> (abs(x)=w415:dbl)
                                n271 = local write "Diferença em %"(w415) -> ()
                                n272 = Divide(x=w415, y=w416) -> (x/y=w418:dbl)
                                n273 = Round To Nearest(number=w418) -> (nearest integer value=w419:dbl)
                                n274 = local write "Quantidade de Passos"(w419) -> ()
                                }
                                frame #1 {
                                n275 = local read "Quantidade de Passos"() -> (w422:sgl)
                                n276 = Greater Or Equal?(x=w422, y=sgl 183.0) -> (x >= y?=w420:bool)
                                n277 = case shown="False" w420 {
                                frame False {
                                n278 = local read "Quantidade de Passos"() -> (w424:sgl)
                                n279 = local write "Quantidade de Passos"(w424) -> ()
                                }
                                frame True {
                                n280 = local write "Quantidade de Passos"(sgl 183.0 ("Quantidade de Passos")) -> ()
                                }
                                }
                                }
                                frame #2 {
                                w427 = u16 10 items=["1.0"=10, "1.5"=15, "2.0"=20] ("stop bits (10: 1 bit)")
                                (unwired) u16 10 ("data bits (8)")
                                # "CONFIGURAÇÃO \nCOM PIC"
                                n281 = local read "COM PIC"() -> (w429:refnum<visa-resource-name>)
                                n282 = call-poly "VISA Configure Serial Port"("VISA resource name"=w429, "timeout (10sec)"=u32 120000, "Enable Termination\nChar (T)"=TRUE, "baud rate (9600)"=u32 9600, "parity (0:none)"=enum16{"None", "Odd", "Even", "Mark", "Space"}."None", "stop bits (10: 1 bit)"=w427) -> ("VISA resource name out"=w428:refnum<visa-resource-name>, "error out"=w426:errorcluster)  [unwired: 8 in]
                                n283 = local write "Erro comando PIC"(w426) -> ()
                                }
                                frame #3 {
                                # "AJUSTE GROSSO"
                                n284 = Greater Than 0?(x=w437) -> (x > 0?=w438:bool)
                                n285 = case shown="True" w438 {
                                tunnel: w436 -> [w442 w466]
                                tunnel: w435 -> [w441 w467]
                                frame False {
                                n286 = stacked-sequence {
                                tunnel: [_ _ w463] -> w444
                                frame #0 {
                                n287 = local read "Quantidade de Passos"() -> (w445:sgl)
                                n288 = Format Into String(format string="%d", w445) -> (resulting string=w447:string)  [unwired: 2 in, 1 out]
                                n289 = String Length(string=w447) -> (length=w448:i32)
                                n290 = case shown="1, Default" w448 {
                                tunnel: w447 -> [w450 w453 w455 w458]
                                frame 1, Default {
                                n291 = Concatenate Strings("000" ("string"), w450) -> (w451:string)
                                n292 = local write "N_passos string"(w451) -> ()
                                }
                                frame 2 {
                                n293 = Concatenate Strings("00" ("string"), w453) -> (w452:string)
                                n294 = local write "N_passos string"(w452) -> ()
                                }
                                frame 3 {
                                n295 = Concatenate Strings("0" ("string"), w455) -> (w456:string)
                                n296 = local write "N_passos string"(w456) -> ()
                                }
                                frame 4 {
                                n297 = local write "N_passos string"(w458) -> ()
                                }
                                }
                                }
                                frame #1 {
                                # "adicionar letra"
                                n298 = local read "N_passos string"() -> (w460:string)
                                n299 = Concatenate Strings("D" ("string"), w460, "OK" ("string")) -> (w462:string)
                                n300 = local write "N_passos string"(w462) -> ()
                                }
                                frame #2 {
                                n301 = local read "N_passos string"() -> (w463:string)
                                }
                                }
                                n302 = VISA Write(VISA resource name=w442, write buffer=w444, error in (no error)=w441) -> (VISA resource name out=w440:refnum<visa-resource-name>, return count=w443:u32, error out=w439:errorcluster)
                                n303 = local write "Erro comando PIC"(w439) -> ()
                                n304 = local write "return count"(w443) -> ()
                                n305 = VISA Close(VISA resource name=w440, error in (no error)=w439) -> ()  [unwired: 1 out]
                                }
                                frame True {
                                n306 = stacked-sequence {
                                tunnel: [_ _ w488] -> w469
                                frame #0 {
                                n307 = local read "Quantidade de Passos"() -> (w470:sgl)
                                n308 = Format Into String(format string="%d", w470) -> (resulting string=w472:string)  [unwired: 2 in, 1 out]
                                n309 = String Length(string=w472) -> (length=w473:i32)
                                n310 = case shown="3" w473 {
                                tunnel: w472 -> [w474 w478 w480 w483]
                                frame 1, Default {
                                n311 = Concatenate Strings("000" ("string"), w474) -> (w476:string)
                                n312 = local write "N_passos string"(w476) -> ()
                                }
                                frame 2 {
                                n313 = Concatenate Strings("00" ("string"), w478) -> (w477:string)
                                n314 = local write "N_passos string"(w477) -> ()
                                }
                                frame 3 {
                                n315 = Concatenate Strings("0" ("string"), w480) -> (w481:string)
                                n316 = local write "N_passos string"(w481) -> ()
                                }
                                frame 4 {
                                n317 = local write "N_passos string"(w483) -> ()
                                }
                                }
                                }
                                frame #1 {
                                n318 = local read "N_passos string"() -> (w485:string)
                                n319 = Concatenate Strings("I" ("string"), w485, "OK" ("string")) -> (w487:string)
                                n320 = local write "N_passos string"(w487) -> ()
                                }
                                frame #2 {
                                n321 = local read "N_passos string"() -> (w488:string)
                                }
                                }
                                n322 = VISA Write(VISA resource name=w466, write buffer=w469, error in (no error)=w467) -> (VISA resource name out=w465:refnum<visa-resource-name>, return count=w468:u32, error out=w464:errorcluster)
                                n323 = local write "Erro comando PIC"(w464) -> ()
                                n324 = local write "return count"(w468) -> ()
                                n325 = VISA Close(VISA resource name=w465, error in (no error)=w464) -> ()  [unwired: 1 out]
                                }
                                }
                                }
                                frame #4 {
                                n326 = Wait (ms)(milliseconds to wait=3000) -> ()  [unwired: 1 out]
                                }
                              }
                              n327 = local write "Motor Disco"(TRUE) -> ()
                            }
                          }
                        }
                      }
                    }
                    frame #2 {
                      n328 = local read "Diferença em %"() -> (w492:dbl)
                      n329 = local write "Ajuste Grosso"(TRUE ("Ajuste Grosso")) -> ()
                      n330 = Multiply(x=w492, y=100.0) -> (x*y=w490:dbl)
                      n331 = Less?(x=w490, y=5) -> (x < y?=w494:bool)
                    }
                  }
                  n332 = local write "Motor Sensor"(FALSE ("Motor Sensor")) -> ()
                  "i" <- w252
                }
              }
              frame #3 {
                n333 = flat-sequence {
                  tunnel: [w503] -> w499
                  tunnel: [w502] -> w498
                  tunnel: w499 -> [w511]
                  tunnel: w498 -> [w510]
                  frame #0 {
                    w501 = u16 10 items=["1.0"=10, "1.5"=15, "2.0"=20] ("stop bits (10: 1 bit)")
                    (unwired) u8 13 ("termination char\n(0xA = '\\n' = LF)")
                    (unwired) u16 10 ("data bits (8)")
                    # "CONFIGURAÇÃO COMUNICAÇÃO PIC"
                    n334 = local read "COM PIC"() -> (w508:refnum<visa-resource-name>)
                    n335 = local write "i"(0 ("i")) -> ()
                    n336 = call-poly "VISA Configure Serial Port"("VISA resource name"=w508, "timeout (10sec)"=u32 120000, "Enable Termination\nChar (T)"=TRUE, "baud rate (9600)"=u32 9600, "parity (0:none)"=enum16{"None", "Odd", "Even", "Mark", "Space"}."None", "stop bits (10: 1 bit)"=w501) -> ("VISA resource name out"=w503:refnum<visa-resource-name>, "error out"=w502:errorcluster)  [unwired: 8 in]
                  }
                  frame #1 {
                    n337 = Wait (ms)(milliseconds to wait=u32 1500) -> ()  [unwired: 1 out]
                    n338 = while {
                      tunnel: w511 -> [w514]
                      tunnel: w510 -> [w513]
                      stop <- w512 stop-if-true
                      n339 = stacked-sequence {
                        tunnel: w514 -> [_ w553]
                        tunnel: w513 -> [_ w552]
                        tunnel: [_ w547] -> w512
                        frame #0 {
                          n340 = disable-structure shown="Enabled" {
                            frame Enabled {
                              n341 = stacked-sequence {
                                frame #0 {
                                n342 = Wait (ms)(milliseconds to wait=u32 1000) -> ()  [unwired: 1 out]
                                }
                                frame #1 {
                                # "AMOSTRAGEM (1 VALOR)"
                                n343 = call "Connect_To_Meter.vi"("Location of FieldMax2Lib.dll in"="Location of FieldMax2Lib.dll in 4") -> ("Meter Serial Number"=→"Meter Serial Number 4":string, "Meter ID out"=w525:i32, "Location of FieldMax2Lib.dll out"=w524:path)  [unwired: 6 in]
                                n344 = dll-call lib="C:/Windows/System32/FieldMax2Lib.dll" fn="fm2LibSync" label="Sync"(path in=w524, "h"=w525) -> (path out=w526:path, "h"=w527:i32)  [unwired: 3 in, 1 out]
                                n345 = Initialize Array(u8 0 ("element"), 64 ("dimension size")) -> (w518:u8[])
                                n346 = while {
                                tunnel: w527 -> [w529]
                                tunnel: w518 -> [w535]
                                tunnel: i16 8 ("count") -> [w534]
                                tunnel: [w531] -> w522
                                tunnel: w526 -> [w536]
                                tunnel: [w530] -> w523
                                stop <- w528 stop-if-true
                                n347 = dll-call lib="C:/Windows/System32/FieldMax2Lib.dll" fn="fm2LibGetData" label="Get Data"(path in=w536, "h"=w529, "returnBuffer"=w535, "count"=w534) -> (path out=w530:path, "h"=w531:i32, "returnBuffer"=w532:u8[], "count"=w533:i16)  [unwired: 3 in, 1 out]
                                n348 = Not Equal To 0?(x=w533) -> (x != 0?=w537:bool)
                                n349 = call "Utility - Bytes to Values.vi"("DataBuffer"=w532) -> ("Measurement Value"=w538:sgl)  [unwired: 9 in, 1 out]
                                n350 = Wait (ms)(milliseconds to wait=u32 1000) -> ()  [unwired: 1 out]
                                n351 = case shown="True" w537 {
                                tunnel: w538 -> [_ w542]
                                tunnel: [FALSE TRUE] -> w528
                                frame False {
                                }
                                frame True {
                                n352 = local write "Measurement (W)"(w542) -> ()
                                }
                                }
                                }
                                n353 = call "Disconnect_From_Meter.vi"("Location of FieldMax2Lib.dll in"=w523, "Meter ID in"=w522) -> ()  [unwired: 7 in, 2 out]
                                }
                              }
                            }
                            frame Disabled {
                              n354 = flat-sequence {
                                frame #0 {
                                n355 = Wait (ms)(milliseconds to wait=u32 500) -> ()  [unwired: 1 out]
                                }
                                frame #1 {
                                n356 = local write "Measurement (W)"(0.145 ("Measurement")) -> ()
                                }
                              }
                            }
                          }
                        }
                        frame #1 {
                          n357 = local read "Setpoint (W)"() -> (w550:dbl)
                          n358 = local read "Measurement (W)"() -> (w551:dbl)
                          n359 = Subtract(x=w550, y=w551) -> (x-y=w546:dbl)
                          n360 = Absolute Value(x=w546) -> (abs(x)=w545:dbl)
                          n361 = Less?(x=w545, y=0.0004) -> (x < y?=w548:bool)
                          n362 = case shown="False" w548 {
                            tunnel: w553 -> [w560 _]
                            tunnel: w552 -> [w554 _]
                            tunnel: [FALSE TRUE] -> w547
                            frame False {
                              # "AJUSTE FINO"
                              n363 = local read "Measurement (W)"() -> (w557:dbl)
                              n364 = local read "Setpoint (W)"() -> (w556:dbl)
                              n365 = local write "Erro comando PIC"(w554) -> ()
                              n366 = local write "Motor Disco"(TRUE) -> ()
                              n367 = Greater?(x=w556, y=w557) -> (0:w559:bool)
                              n368 = case shown="True" w559 {
                                tunnel: w556 -> [w565 _]
                                tunnel: w557 -> [w564 _]
                                tunnel: w560 -> [w562 w579]
                                tunnel: w554 -> [w561 w578]
                                frame False {
                                n369 = Equal?(x=w565, y=w564) -> (x = y?=w563:bool)
                                n370 = case shown="False" w563 {
                                tunnel: w562 -> [w568 w574]
                                tunnel: w561 -> [w567 w573]
                                frame False {
                                n371 = VISA Write(VISA resource name=w568, write buffer="D0001OK", error in (no error)=w567) -> (return count=w569:u32, error out=w566:errorcluster)  [unwired: 1 out]
                                n372 = local write "Erro comando PIC"(w566) -> ()
                                n373 = local write "return count"(w569) -> ()
                                }
                                frame True {
                                n374 = VISA Write(VISA resource name=w574, write buffer="S0000OK", error in (no error)=w573) -> (VISA resource name out=w572:refnum<visa-resource-name>, return count=w575:u32, error out=w571:errorcluster)
                                n375 = local write "return count"(w575) -> ()
                                n376 = local write "Erro comando PIC"(w571) -> ()
                                n377 = VISA Close(VISA resource name=w572, error in (no error)=w571) -> ()  [unwired: 1 out]
                                }
                                }
                                }
                                frame True {
                                n378 = VISA Write(VISA resource name=w579, write buffer="I0001OK", error in (no error)=w578) -> (return count=w580:u32, error out=w577:errorcluster)  [unwired: 1 out]
                                n379 = local write "Erro comando PIC"(w577) -> ()
                                n380 = local write "return count"(w580) -> ()
                                }
                              }
                            }
                            frame True {
                            }
                          }
                        }
                      }
                    }
                  }
                }
                n381 = local write "Ajuste Fino"(TRUE ("Ajuste Fino")) -> ()
                n382 = local write "Ajuste Grosso"(FALSE ("Ajuste Grosso")) -> ()
              }
              frame #4 {
                n383 = stacked-sequence {
                  frame #0 {
                    n384 = Wait (ms)(milliseconds to wait=u32 500) -> ()  [unwired: 1 out]
                  }
                  frame #1 {
                    n385 = disable-structure shown="Enabled" {
                      frame Enabled {
                        # "AMOSTRAGEM (1 VALOR)"
                        n386 = call "Connect_To_Meter.vi"("Location of FieldMax2Lib.dll in"="Location of FieldMax2Lib.dll in 5") -> ("Meter Serial Number"=→"Meter Serial Number 5":string, "Meter ID out"=w594:i32, "Location of FieldMax2Lib.dll out"=w593:path)  [unwired: 6 in]
                        n387 = dll-call lib="C:/Windows/System32/FieldMax2Lib.dll" fn="fm2LibSync" label="Sync"(path in=w593, "h"=w594) -> (path out=w595:path, "h"=w596:i32)  [unwired: 3 in, 1 out]
                        n388 = Initialize Array(u8 0 ("element"), 64 ("dimension size")) -> (w587:u8[])
                        n389 = while {
                          tunnel: w596 -> [w598]
                          tunnel: w587 -> [w604]
                          tunnel: i16 8 ("count") -> [w603]
                          tunnel: [w600] -> w591
                          tunnel: w595 -> [w605]
                          tunnel: [w599] -> w592
                          stop <- w597 stop-if-true
                          n390 = dll-call lib="C:/Windows/System32/FieldMax2Lib.dll" fn="fm2LibGetData" label="Get Data"(path in=w605, "h"=w598, "returnBuffer"=w604, "count"=w603) -> (path out=w599:path, "h"=w600:i32, "returnBuffer"=w601:u8[], "count"=w602:i16)  [unwired: 3 in, 1 out]
                          n391 = Not Equal To 0?(x=w602) -> (x != 0?=w606:bool)
                          n392 = call "Utility - Bytes to Values.vi"("DataBuffer"=w601) -> ("Measurement Value"=w607:sgl)  [unwired: 9 in, 1 out]
                          n393 = Wait (ms)(milliseconds to wait=u32 1000) -> ()  [unwired: 1 out]
                          n394 = case shown="True" w606 {
                            tunnel: w607 -> [_ w611]
                            tunnel: [FALSE TRUE] -> w597
                            frame False {
                            }
                            frame True {
                              n395 = local write "Measurement (W)"(w611) -> ()
                            }
                          }
                        }
                        n396 = call "Disconnect_From_Meter.vi"("Location of FieldMax2Lib.dll in"=w592, "Meter ID in"=w591) -> ()  [unwired: 7 in, 2 out]
                      }
                      frame Disabled {
                        n397 = local write "Measurement (W)"(0.1159) -> ()
                      }
                    }
                  }
                  frame #2 {
                    n398 = flat-sequence {
                      frame #0 {
                        n399 = local read "Measurement (W)"() -> (w616:dbl)
                        n400 = Number To Fractional String(number=w616, precision (6)=i16 4) -> (F-format string=w617:string)  [unwired: 2 in]
                        n401 = Scan From String(format string="%6.4f", input string=w617) -> (output 1=w613:dbl)  [unwired: 3 in, 3 out]
                        n402 = Format Into String(format string="%6.4f", w613) -> (resulting string=w614:string)  [unwired: 2 in, 1 out]
                        n403 = local write "Resulting string (W)"(w614) -> ()
                      }
                      frame #1 {
                        n404 = local read "Resulting string (W)"() -> (w622:string)
                        n405 = Concatenate Strings("Potencia_ajustada:", w622) -> (w620:string)
                        n406 = local write "Resulting string (W)"(w620) -> ()
                      }
                    }
                  }
                }
                n407 = local write "Ajuste Fino"(FALSE ("Ajuste Fino")) -> ()
              }
              frame #5 {
                n408 = flat-sequence {
                  tunnel: [w636] -> w632
                  tunnel: [w634] -> w631
                  tunnel: w632 -> [w645]
                  tunnel: w631 -> [w644]
                  tunnel: [w643] -> w626
                  tunnel: [w642] -> w624
                  tunnel: w626 -> [w652]
                  tunnel: [w652] -> w625
                  tunnel: w624 -> [w651]
                  tunnel: [w651] -> w623
                  tunnel: w625 -> [w656]
                  tunnel: w623 -> [w655]
                  tunnel: [w654] -> w630
                  tunnel: [w653] -> w628
                  tunnel: w630 -> [w663]
                  tunnel: [w663] -> w629
                  tunnel: w628 -> [w662]
                  tunnel: [w662] -> w627
                  tunnel: w629 -> [w667]
                  tunnel: w627 -> [w666]
                  frame #0 {
                    n409 = Wait (ms)(milliseconds to wait=u32 3000) -> ()  [unwired: 1 out]
                  }
                  frame #1 {
                    w635 = u16 10 items=["1.0"=10, "1.5"=15, "2.0"=20] ("stop bits (10: 1 bit)")
                    (unwired) u8 13 ("termination char\n(0xA = '\\n' = LF)")
                    (unwired) u16 10 ("data bits (8)")
                    # "CONFIGURAÇÃO COMUNICAÇÃO PIC"
                    n410 = local read "COM PIC"() -> (w641:refnum<visa-resource-name>)
                    n411 = call-poly "VISA Configure Serial Port"("VISA resource name"=w641, "timeout (10sec)"=u32 120000, "Enable Termination\nChar (T)"=TRUE, "baud rate (9600)"=u32 9600, "parity (0:none)"=enum16{"None", "Odd", "Even", "Mark", "Space"}."None", "stop bits (10: 1 bit)"=w635) -> ("VISA resource name out"=w636:refnum<visa-resource-name>, "error out"=w634:errorcluster)  [unwired: 8 in]
                    n412 = local write "Erro comando PIC"(w634) -> ()
                  }
                  frame #2 {
                    # "FECHAMENTO OBTURADOR"
                    n413 = local write "Shutter ON (Verde_Claro)/ OFF (Verde_Escuro)"(TRUE ("Inicia Controle")) -> ()
                    n414 = VISA Write(VISA resource name=w645, write buffer="F0000OK", error in (no error)=w644) -> (VISA resource name out=w643:refnum<visa-resource-name>, return count=w649:u32, error out=w642:errorcluster)
                    n415 = local write "return count"(w649) -> ()
                    n416 = local write "Motor Disco"(FALSE) -> ()
                    n417 = local write "Erro comando PIC"(w642) -> ()
                  }
                  frame #3 {
                    n418 = Wait (ms)(milliseconds to wait=u32 1000) -> ()  [unwired: 1 out]
                  }
                  frame #4 {
                    # "RETIRADA DO SENSOR"
                    n419 = local write "Shutter ON (Verde_Claro)/ OFF (Verde_Escuro)"(TRUE) -> ()
                    n420 = VISA Write(VISA resource name=w656, write buffer="R0000OK", error in (no error)=w655) -> (VISA resource name out=w654:refnum<visa-resource-name>, return count=w657:u32, error out=w653:errorcluster)
                    n421 = local write "return count"(w657) -> ()
                    n422 = local write "Erro comando PIC"(w653) -> ()
                    n423 = local write "Motor Sensor"(TRUE) -> ()
                  }
                  frame #5 {
                    n424 = Wait (ms)(milliseconds to wait=u32 2500) -> ()  [unwired: 1 out]
                  }
                  frame #6 {
                    # "FECHAMENTO DO OBTURADOR"
                    n425 = local write "Shutter ON (Verde_Claro)/ OFF (Verde_Escuro)"(FALSE) -> ()
                    n426 = local write "Motor Sensor"(FALSE) -> ()
                    n427 = VISA Write(VISA resource name=w667, write buffer="F0000OK", error in (no error)=w666) -> (VISA resource name out=w665:refnum<visa-resource-name>, return count=w672:u32, error out=w664:errorcluster)
                    n428 = local write "return count"(w672) -> ()
                    n429 = property on="Setpoint (W)" class="DigNum (strict)"("DisabledEnum"=T2."Enabled" ("Disabled")) -> ()  [unwired: 2 in, 2 out]
                    n430 = VISA Close(VISA resource name=w665, error in (no error)=w664) -> ()  [unwired: 1 out]
                  }
                }
              }
              frame #6 {
                # "potencia_ajustada:0,0000(24caracteres)"
                # "AVISO AO USUÁRIO DE POTÊNCIA AJUSTADA"
                n431 = flat-sequence {
                  frame #0 {
                    n432 = local read "connection P3D ID out"() -> (w675:refnum<k5>)
                    n433 = local read "Erro TCP 3DP"() -> (w676:errorcluster)
                    n434 = while {
                      tunnel: [w686] -> w674
                      tunnel: [w684] -> _
                      tunnel: w675 -> [w678]
                      tunnel: w676 -> [w677]
                      stop <- w683 stop-if-true
                      n435 = local read "Resulting string (W)"() -> (w679:string)
                      n436 = TCP Write(connection ID=w678, data in=w679, error in (no error)=w677) -> (connection ID out=w686:refnum<k5>, bytes written=w682:i32, error out=w684:errorcluster)  [unwired: 1 in]
                      n437 = Unbundle By Name(w684) -> ("status"=w685:bool)
                      n438 = Equal?(x=w682, y=24) -> (x = y?=w680:bool)
                      n439 = Or(x=w685, y=w680) -> (x .or. y?=w683:bool)
                    }
                    n440 = local write "connection P3D ID out"(w674) -> ()
                  }
                  frame #1 {
                    n441 = Wait (ms)(milliseconds to wait=u32 1000) -> ()  [unwired: 1 out]
                  }
                }
              }
            }
          }
          frame "Stop" {
            n442 = flat-sequence {
              frame #0 {
                n443 = local read "COM PIC"() -> (w698:refnum<visa-resource-name>)
                n444 = call-poly "VISA Configure Serial Port"("VISA resource name"=w698, "timeout (10sec)"=u32 10000, "termination char\n(0xA = '\\n' = LF)"=u8 10 ("termination char\n(0xA = '\\n' = LF)"), "Enable Termination\nChar (T)"=FALSE ("Enable Termination\nChar (T)"), "baud rate (9600)"=u32 9600, "data bits (8)"=u16 8, "parity (0:none)"=enum16{"None", "Odd", "Even", "Mark", "Space"}."None") -> ("VISA resource name out"=w694:refnum<visa-resource-name>, "error out"=w693:errorcluster)  [unwired: 7 in]
                n445 = VISA Write(VISA resource name=w694, write buffer="F0000OK", error in (no error)=w693) -> (VISA resource name out=w692:refnum<visa-resource-name>, error out=w691:errorcluster)  [unwired: 1 out]
                n446 = local write "Shutter ON (Verde_Claro)/ OFF (Verde_Escuro)"(TRUE ("Inicia Controle")) -> ()
                n447 = VISA Write(VISA resource name=w692, write buffer="S0000OK", error in (no error)=w691) -> (VISA resource name out=w696:refnum<visa-resource-name>, return count=w695:u32, error out=w697:errorcluster)
                n448 = local write "return count"(w695) -> ()
                n449 = local write "Motor Sensor"(TRUE) -> ()
                n450 = VISA Close(VISA resource name=w696, error in (no error)=w697) -> ()  [unwired: 1 out]
              }
              frame #1 {
                n451 = local write "Mensagem de erro renviada"("Ops! Algo deu errado...") -> ()
              }
              frame #2 {
                n452 = local read "connection P3D ID out"() -> (w710:refnum<k5>)
                n453 = local read "Erro TCP 3DP"() -> (w711:errorcluster)
                n454 = TCP Write(connection ID=w710, data in="Mensagem de erro renviada", error in (no error)=w711) -> ()  [unwired: 1 in, 3 out]
              }
            }
            n455 = property on="Setpoint (W)" class="DigNum (strict)"("DisabledEnum"=T2."Disabled" ("Disabled")) -> ()  [unwired: 2 in, 2 out]
          }
        }
      }
      event "Quit": Value Change {
        w712 = "Encerra Programa?" ("message")
        n456 = event-data() -> ()  [unwired: 1 in, 5 out]
        n457 = local write "Mensagem de erro renviada"(w712) -> ()
        n458 = Two Button Dialog(message=w712, 1:"Não" ("F button name (\"Cancel\")"), 2:"Sim" ("T button name (\"OK\")")) -> (T button?=w718:bool)
        n459 = Select(t=TCC_01_02_15."Stop", s=w718, f=TCC_01_02_15."Receber Potencia") -> (s? t:f=w713:T1)
      }
      event "Erro comando PIC": Value Change {
        n460 = event-data() -> ()  [unwired: 1 in, 5 out]
      }
    }
    n461 = Equal?(x=w5, y=TCC_01_02_15."Stop" ("States")) -> (x = y?=w7:bool)
    n462 = Wait (ms)(milliseconds to wait=u32 125) -> ()  [unwired: 1 out]
  }
